vi "CLD 12 File Commands Utility.vi"(7 "Error In":errorcluster) -> (2 "Error Out":errorcluster, 3 "Commands Out Array":T1[](array[typedef]))   [LabVIEW 2018]
uses:
  CLD 12 Data Cluster.ctl
  CLD 12 Sequencer Enum.ctl
  <vilib>/Utility/file.llb/Read Delimited Spreadsheet (string).vi
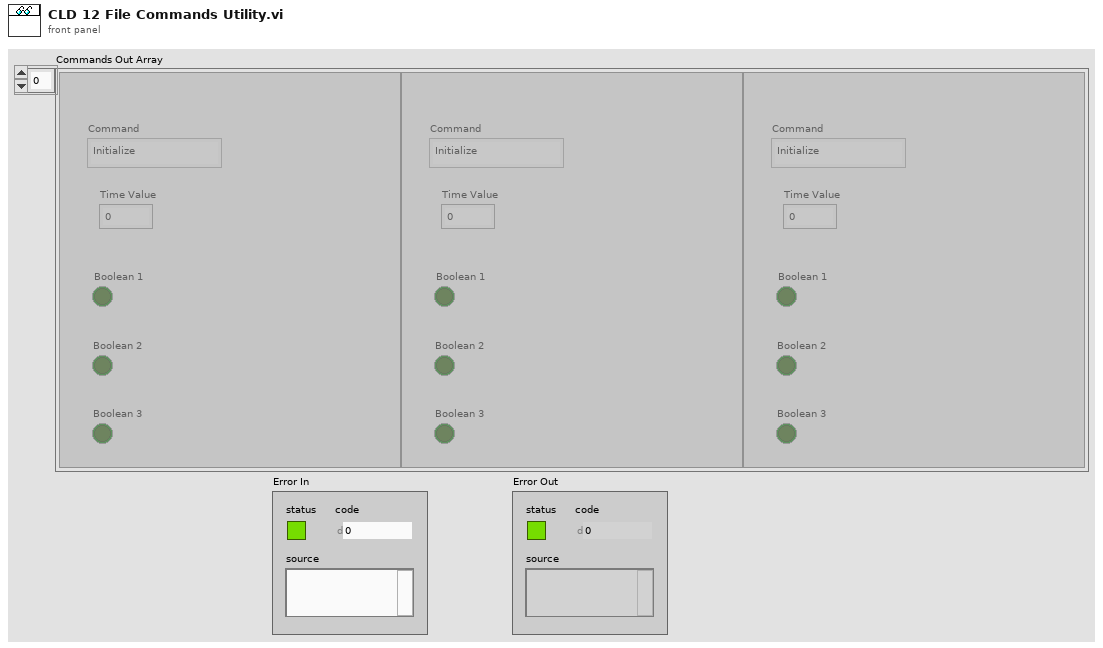
[diagram p1: front panel]
types:
  T1 = typedef "CLD 12 Data Cluster.ctl" = cluster{"Command":T2, "Time Value":dbl, "Boolean 1":bool, "Boolean 2":bool, "Boolean 3":bool}
  T2 = typedef "CLD 12 Sequencer Enum.ctl" = enum16{"Initialize", "SetTime", "RunState1", "Runstate2", "Idle", "Start"}
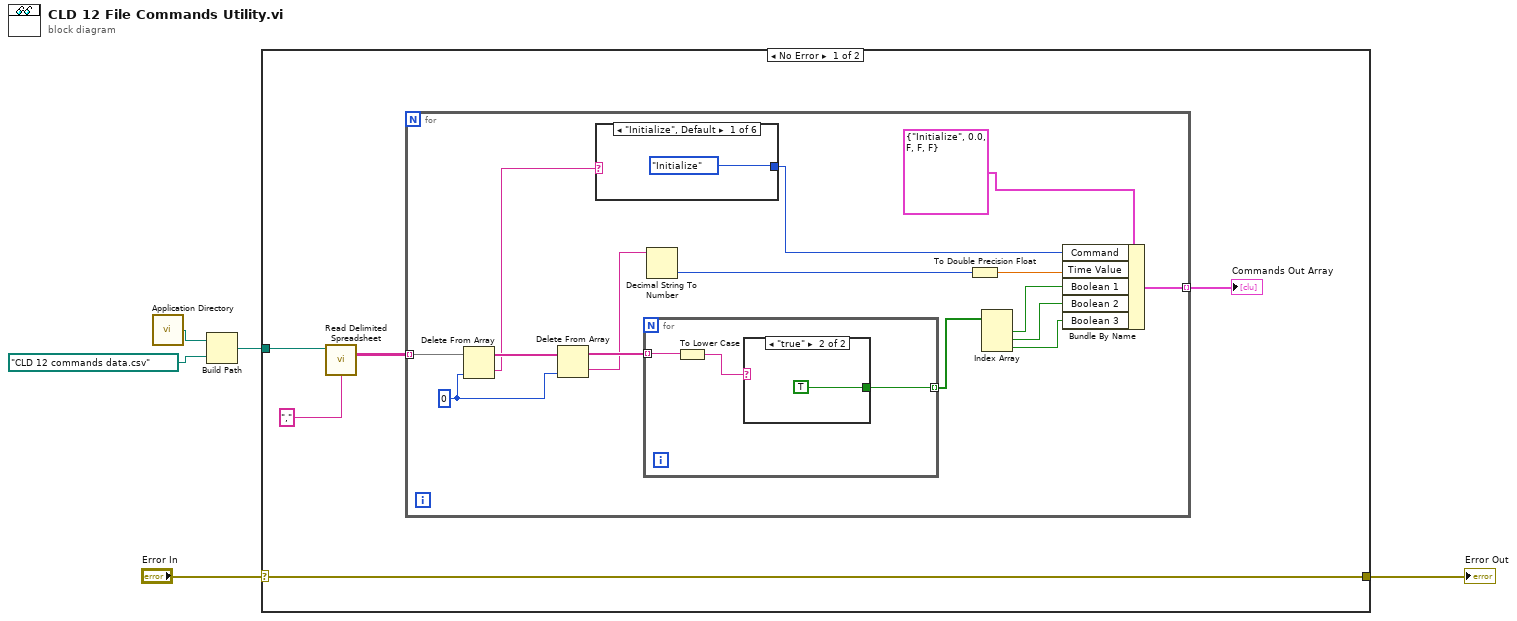
[diagram p0: block diagram]
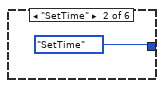
[diagram p2: hidden frame]
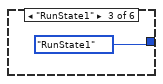
[diagram p3: hidden frame]
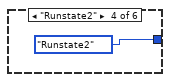
[diagram p4: hidden frame]
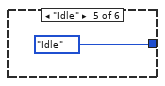
[diagram p5: hidden frame]
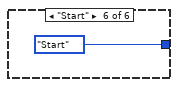
[diagram p6: hidden frame]
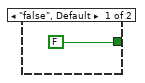
[diagram p7: hidden frame]
diagram:
  n1 = call <vilib>:"Application Directory.vi"() -> ("Application Directory"=w5:path)
  n2 = Build Path(base path=w5, name or relative path=path "CLD 12 commands data.csv") -> (appended path=w4:path)
  n3 = case shown="No Error" "Error In" {
    selector: "Error In" -> [w7 w37]
    tunnel: w4 -> [w10 _]
    tunnel: [w7 w37] -> w2
    frame No Error {
      n4 = call-poly <vilib>:"Read Delimited Spreadsheet.vi"("file path (dialog if empty)"=w10, "delimiter (\\t)"="," ("delimiter (\\t)")) -> ("all rows"=w8:string[][])  [unwired: 8 in, 5 out]
      n5 = for {
        tunnel: w8 -> [w25] mode=indexing
        tunnel: [w11] -> w6 mode=indexing
        w23 = 0 ("index")
        n6 = Delete From Array(array=w25, index=w23) -> (deleted portion=w17:string, array with subset deleted=w24:string[])  [unwired: 1 in]
        n7 = Delete From Array(array=w24, index=w23) -> (deleted portion=w15:string, array with subset deleted=w22:string[])  [unwired: 1 in]
        n8 = case shown="\"Initialize\", Default" w17 {
          tunnel: [CLD_12_Sequencer_Enum."Initialize" ("Command") CLD_12_Sequencer_Enum."SetTime" ("Command") CLD_12_Sequencer_Enum."RunState1" ("Command") CLD_12_Sequencer_Enum."Runstate2" ("Command") CLD_12_Sequencer_Enum."Idle" ("Command") CLD_12_Sequencer_Enum."Start" ("Command")] -> w16
          frame "Initialize", Default {
          }
          frame "SetTime" {
          }
          frame "RunState1" {
          }
          frame "Runstate2" {
          }
          frame "Idle" {
          }
          frame "Start" {
          }
        }
        n9 = for {
          tunnel: w22 -> [w34] mode=indexing
          tunnel: [w32] -> w21 mode=indexing
          n10 = To Lower Case(string=w34) -> (all lower case string=w33:string)
          n11 = case shown="\"true\"" w33 {
            tunnel: [FALSE TRUE] -> w32
            frame "false", Default {
            }
            frame "true" {
            }
          }
        }
        n12 = Decimal String To Number(string=w15) -> (number=w14:i32)  [unwired: 2 in, 1 out]
        n13 = To Double Precision Float(number=w14) -> (double precision float=w13:dbl)
        n14 = Index Array(array=w21) -> (element #1=w20:bool, element #2=w19:bool, element #3=w18:bool)  [unwired: 3 in]
        n15 = Bundle By Name(cluster=T1 {"Command"=enum."Initialize", "Time Value"=0.0, "Boolean 1"=FALSE, "Boolean 2"=FALSE, "Boolean 3"=FALSE} ("CLD 12 Data Cluster"), "Command"=w16, "Time Value"=w13, "Boolean 1"=w20, "Boolean 2"=w19, "Boolean 3"=w18) -> (w11:T1)
      }
      "Commands Out Array" <- w6
    }
    frame Error {
    }
  }
  "Error Out" <- w2
